vi "Create by Path and Filter.vi"(8 "错误输入（无错误）":errorcluster, 10 "filter":string, 11 "Dir Path":path) -> (0 "错误输出":errorcluster, 3 "FileSystem Watcher Ref":refnum<k24>)   [LabVIEW 2012, in "FileSystem Watcher.lvlib"]
uses:
  FileSystem Watcher.lvlib
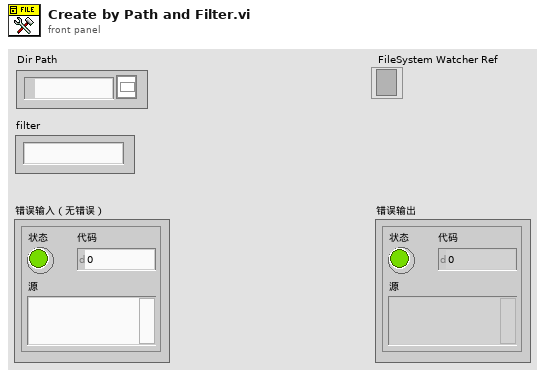
[diagram p1: front panel]
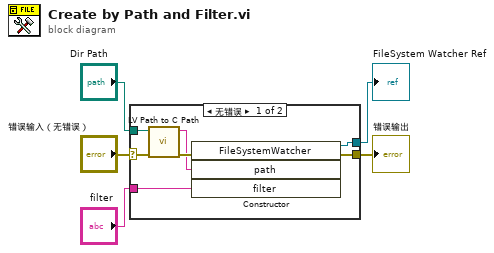
[diagram p0: block diagram]
diagram:
  n1 = case shown="无错误" "错误输入（无错误）" {
    selector: "错误输入（无错误）" -> [w9 w13]
    tunnel: [w12 w13] -> w4
    tunnel: [w11 _] -> w3
    tunnel: "filter" -> [w10 _]
    tunnel: "Dir Path" -> [w7 _]
    frame No Error {
      n2 = call "LV Path to C Path.vi"("错误输入（无错误）"=w9, "Dir Path"=w7) -> ("错误输出"=w8:errorcluster, "C Path"=w6:string)  [unwired: 8 in]
      n3 = constructor class="FileSystemWatcher"(error in=w8, "path"=w6, "filter"=w10) -> (reference out=w11:refnum<k24>, error out=w12:errorcluster)  [unwired: 2 in, 3 out]
    }
    frame Error {
    }
  }
  "错误输出" <- w4
  "FileSystem Watcher Ref" <- w3
